vi "S2DS_ChangeReadFactors.vi"(3 "RC info list (in)":T1) -> (1 "RC info list (out)":T1)   [LabVIEW 2025]
uses:
  TYPE DEFS/S2DS_RC info.ctl
  TYPE DEFS/S2DS_Single RC info.ctl
panel:
  in  "EXIT":bool
  out "Wait (ms) 3":i32
  out "Averaging 3":i32
  out "Factor 3":dbl
  out "Array":string[](array[string])
  in  "Wait (ms) 2":i32
  in  "Averaging 2":i32=1
  in  "Factor 2":dbl=1.0
  out "Wait (ms)":i32
  out "Averaging":i32
  out "Factor":dbl
  in  "select channel to edit":u16(ring)
  in  "Cancel":bool
  in  "OK":bool
  # "Edit reading channel info..."
  # "Parameter name"
  # "Updated"
  # "Enter new"
  # "Old"
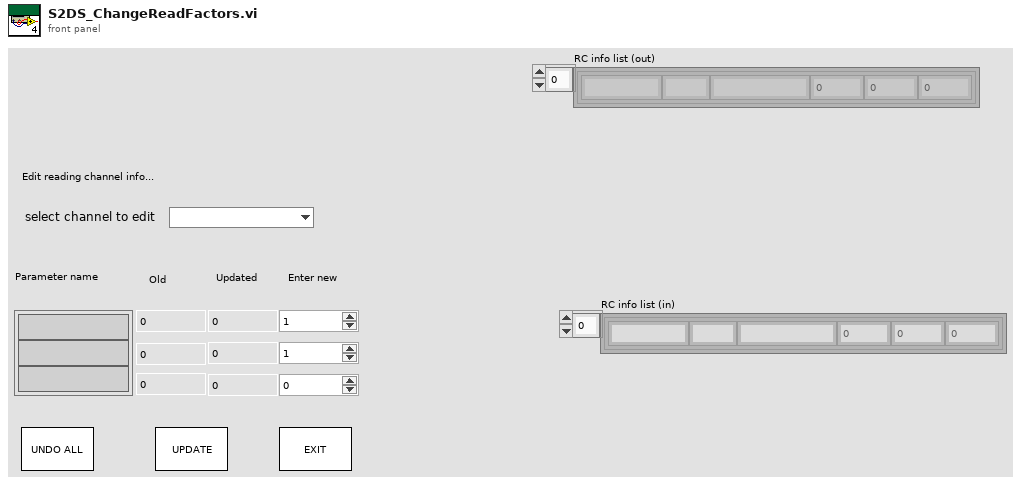
[diagram p1: front panel]
types:
  T1 = typedef "S2DS_RC info.ctl" = T2[]
  T2 = typedef "S2DS_Single RC info.ctl" = cluster{"Instrument identifier":string, "Factor":dbl, "Averaging":i32, "Wait (ms)":i32, "Unit":string, "Name":string}
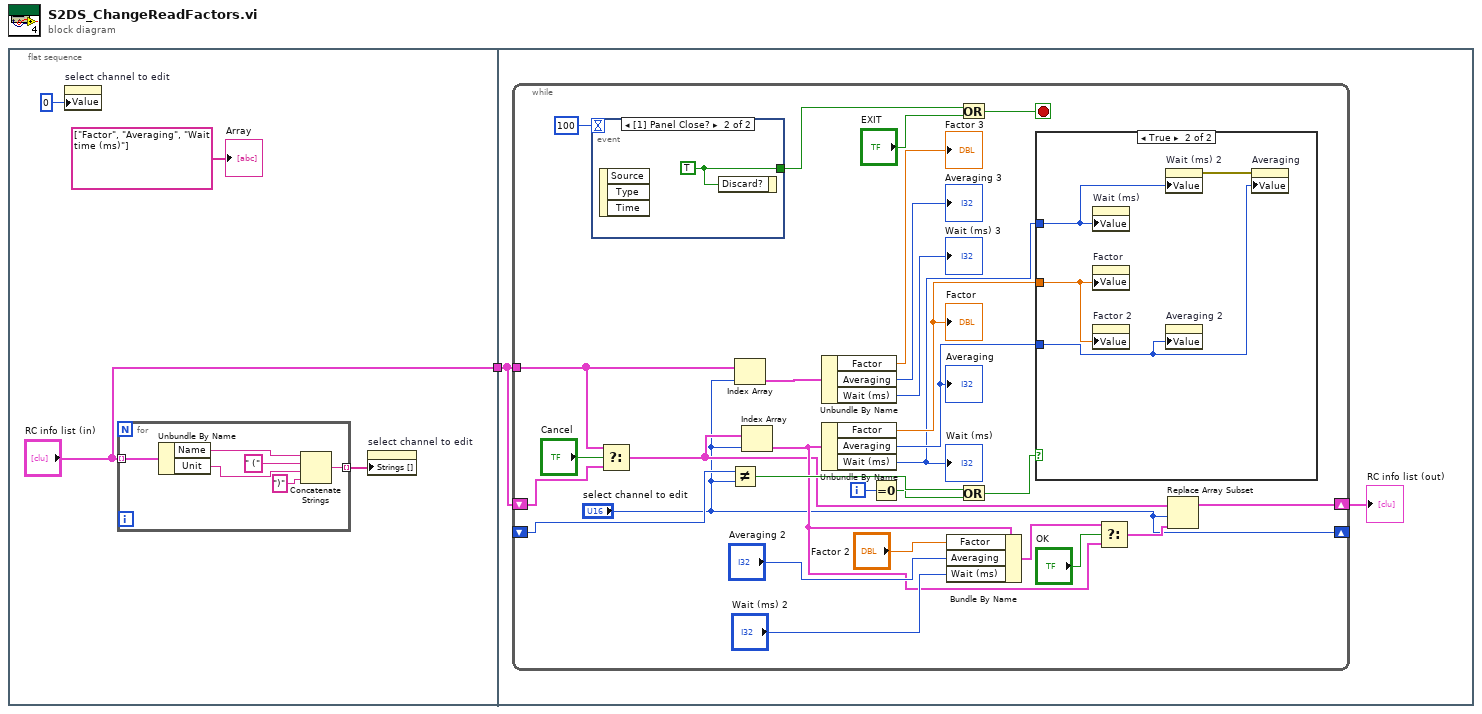
[diagram p0: block diagram]
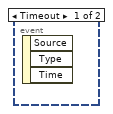
[diagram p2: hidden frame]
diagram:
  n1 = flat-sequence {
    tunnel: ["RC info list (in)"] -> w1
    tunnel: w1 -> [w12]
    frame #0 {
      n2 = property on="select channel to edit" class="Ring (strict)"("Value"=0) -> ()  [unwired: 2 in, 2 out]
      n3 = for {
        tunnel: "RC info list (in)" -> [w11] mode=indexing
        tunnel: [w6] -> w2 mode=indexing
        n4 = Unbundle By Name(w11) -> ("Name"=w10:string, "Unit"=w8:string)
        n5 = Concatenate Strings(w10, " (" ("string"), w8, ")" ("string")) -> (w6:string)
      }
      n6 = property on="select channel to edit" class="Ring (strict)"("Strings []"=w2) -> ()  [unwired: 2 in, 2 out]
      "Array" <- string[] ["Factor", "Averaging", "Wait time (ms)"] ("Array")
    }
    frame #1 {
      n7 = while {
        shift-right: [w27] -> w13
        shift-left: w12 -> [w24]
        shift-right: ["select channel to edit"] -> _
        shift-left: _ -> [w42]
        tunnel: w12 -> [w22]
        i -> [w41]
        stop <- w14 stop-if-true
        n8 = event shown="[1] Panel Close?" {
          selector: _ -> [_ _]
          dyn-events: _ -> [_ _]
          timeout: 100 -> [_ _]
          tunnel: [_ w43] -> w15
          event Timeout {
            n9 = event-data() -> ()  [unwired: 1 in, 3 out]
          }
          event Panel Close? {
            w43 = TRUE ("Discard?")
            n10 = event-data() -> ()  [unwired: 1 in, 3 out]
            n11 = event-data("Discard?"=w43) -> ()  [unwired: 1 in, 1 out]
          }
        }
        n12 = Select(t=w22, s="Cancel", f=w24) -> (s? t:f=w23:T1)
        n13 = Not Equal?(x=w42, y="select channel to edit") -> (x != y?=w40:bool)
        n14 = Index Array(array=w22, index="select channel to edit") -> (element=w20:T2)
        n15 = Index Array(array=w23, index="select channel to edit") -> (element=w29:T2)
        n16 = Unbundle By Name(w20) -> ("Factor"=→"Factor 3":dbl, "Averaging"=→"Averaging 3":i32, "Wait (ms)"=→"Wait (ms) 3":i32)
        n17 = Unbundle By Name(w29) -> ("Factor"=w37:dbl, "Averaging"=w36:i32, "Wait (ms)"=w35:i32)
        "Factor" <- w37
        "Averaging" <- w36
        "Wait (ms)" <- w35
        n18 = Equal To 0?(x=w41) -> (x = 0?=w39:bool)
        n19 = Bundle By Name(cluster=w29, "Factor"="Factor 2", "Averaging"="Averaging 2", "Wait (ms)"="Wait (ms) 2") -> (w30:T2)
        n20 = Or(x=w15, y="EXIT") -> (x .or. y?=w14:bool)
        n21 = Or(x=w40, y=w39) -> (x .or. y?=w38:bool)
        n22 = case shown="True" w38 {
          tunnel: w37 -> [_ w47]
          tunnel: w36 -> [_ w46]
          tunnel: w35 -> [_ w44]
          frame False {
          }
          frame True {
            n23 = property on="Wait (ms)" class="DigNum (strict)"("Value"=w44) -> ()  [unwired: 2 in, 2 out]
            n24 = property on="Factor" class="DigNum (strict)"("Value"=w47) -> ()  [unwired: 2 in, 2 out]
            n25 = property on="Factor 2" class="DigNum (strict)"("Value"=w47) -> ()  [unwired: 2 in, 2 out]
            n26 = property on="Wait (ms) 2" class="DigNum (strict)"("Value"=w44) -> (error out=w45:errorcluster)  [unwired: 2 in, 1 out]
            n27 = property on="Averaging 2" class="DigNum (strict)"("Value"=w46) -> ()  [unwired: 2 in, 2 out]
            n28 = property on="Averaging" class="DigNum (strict)"(error in=w45, "Value"=w46) -> ()  [unwired: 1 in, 2 out]
          }
        }
        n29 = Select(t=w30, s="OK", f=w29) -> (s? t:f=w28:T2)
        n30 = Replace Array Subset(array=w23, new element=w28, index="select channel to edit") -> (w27:T1)
      }
      "RC info list (out)" <- w13
    }
  }
